vi "test_Packet_SimplePipelineResult.vi"(8 "error in (no error)":errorcluster) -> (0 "error out":errorcluster, 3 "Test Passed":bool)   [LabVIEW 2020]
uses:
  PhotonVisionLib/PhotonVisionLib.lvlib
  <vilib>/Rock Robotics/WPI/ThirdParty/JAS_Junk/TrajLib/Trajectory_Library.lvlib
  PhotonVisionLib/TypeDef/TargetCornerType.ctl
  <vilib>/Rock Robotics/WPI/ThirdParty/JAS_Junk/TrajLib/TypeDef/TRANSLATION2D.ctl
  <vilib>/Rock Robotics/WPI/ThirdParty/JAS_Junk/TrajLib/TypeDef/ROTATION2D.ctl
  <vilib>/Rock Robotics/WPI/ThirdParty/JAS_Junk/TrajLib/TypeDef/TRANSFORM2D.ctl
  PhotonVisionLib/TypeDef/PhotonTrackedTargetType.ctl
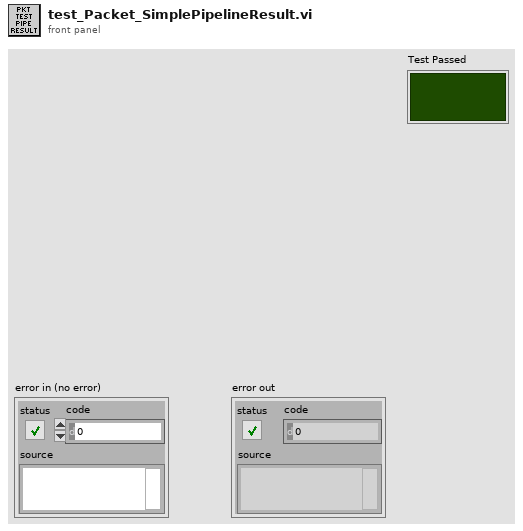
[diagram p1: front panel]
types:
  T1 = typedef "PhotonVisionLib.lvlib/PhotonTrackedTargetType.ctl" = cluster{"Yaw":dbl, "Pitch":dbl, "Area":dbl, "Skew":dbl, "TargetCorners":T2[], "CameraToTarget":T3, "FiducialId":i32}
  T2 = typedef "PhotonVisionLib.lvlib/TargetCornerType.ctl" = cluster{"X":dbl, "Y":dbl}
  T3 = typedef "Trajectory_Library.lvlib/TRANSFORM2D.ctl" = cluster{"TRANSLATION":T4, "ROTATION":T5, "xF":bool}
  T4 = typedef "Trajectory_Library.lvlib/TRANSLATION2D.ctl" = cluster{"X":dbl, "Y":dbl}
  T5 = typedef "Trajectory_Library.lvlib/ROTATION2D.ctl" = cluster{"VALUE":dbl, "COS":dbl, "SIN":dbl}
  T6 = typedef "PhotonVisionLib.lvlib/PhotonPipelineResultType.ctl" = cluster{"TargetCount":i32, "Latency_MilliSec":dbl, "Targets":T1[]}
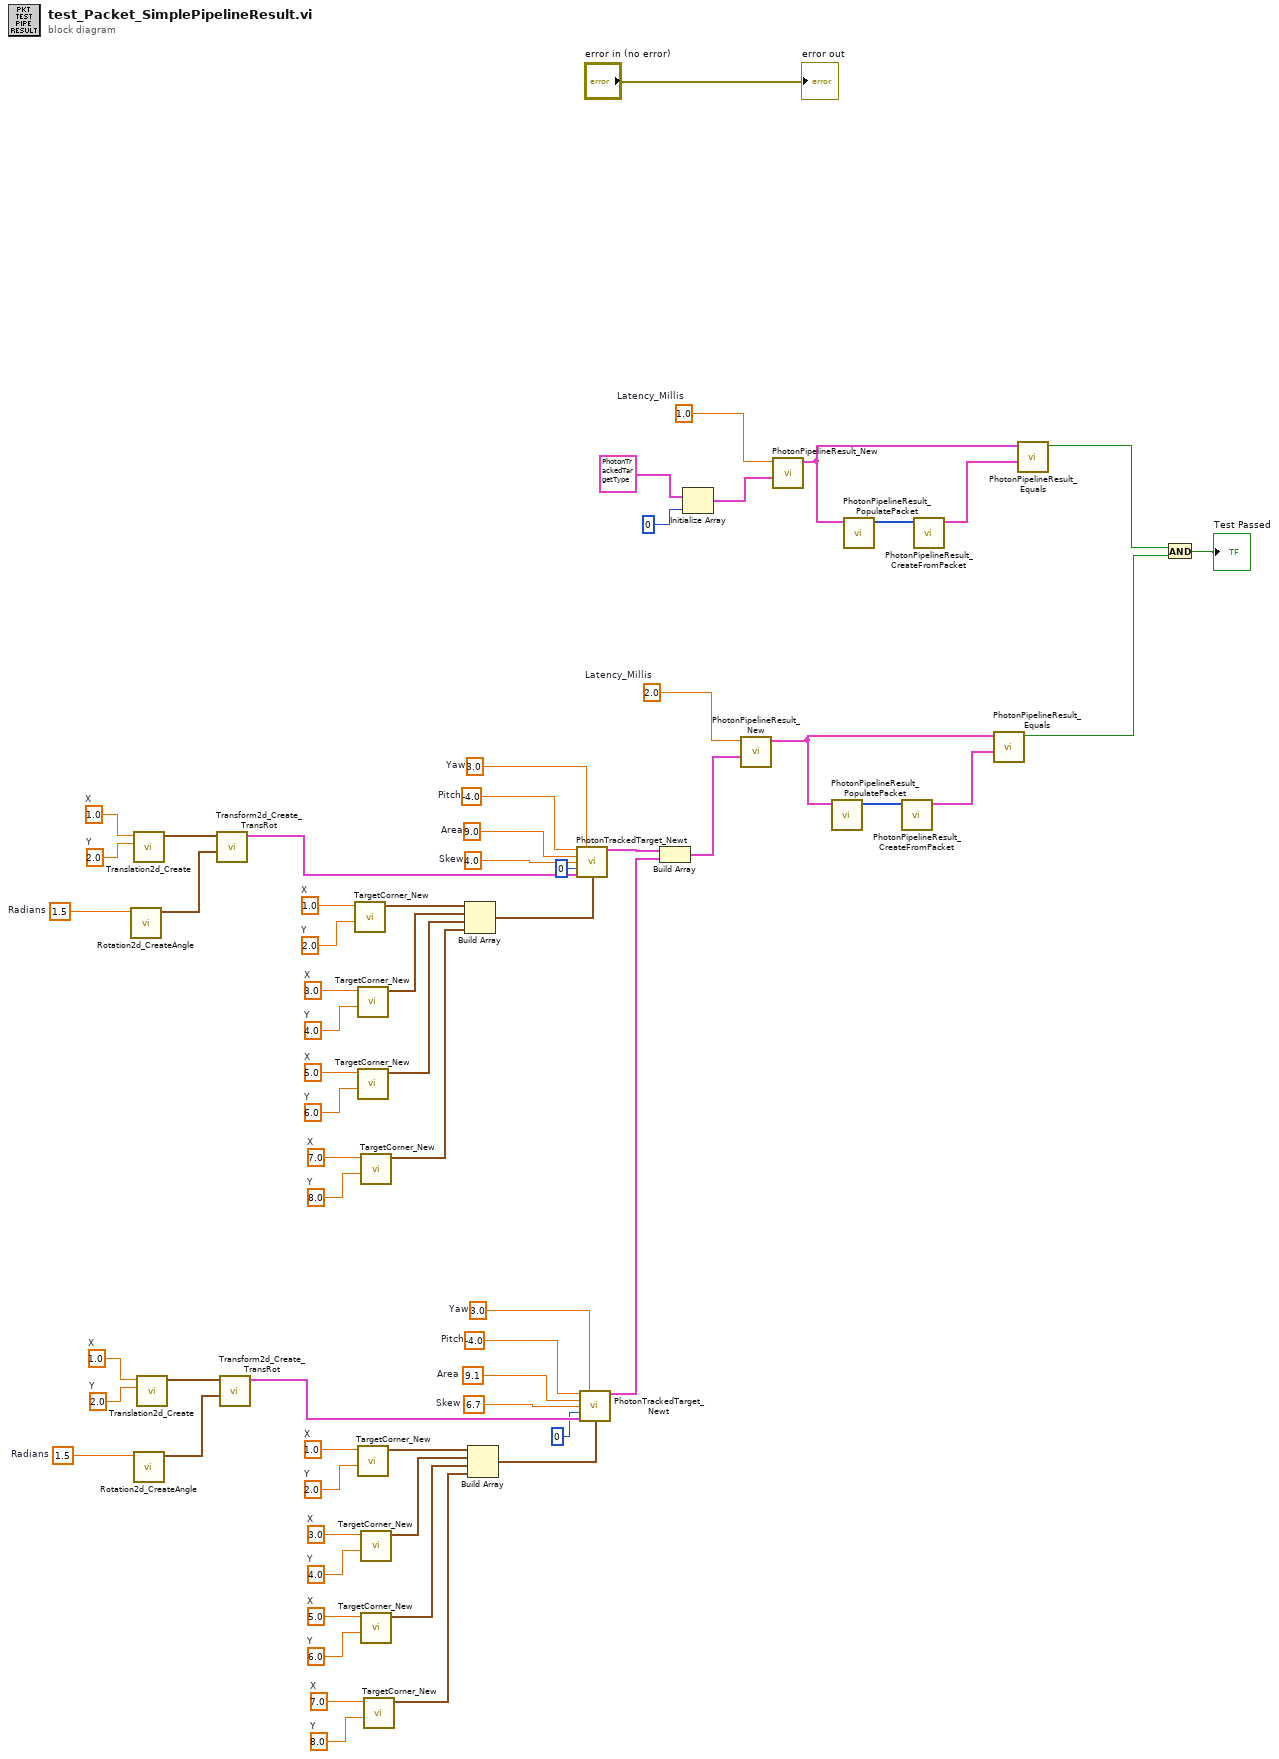
[diagram p0: block diagram]
diagram:
  w14 = 1.0  # Latency_Millis
  w16 = 2.0  # Latency_Millis
  w21 = 1.0  # X
  w22 = 2.0  # Y
  w24 = 1.5  # Radians
  w26 = -4.0  # Pitch
  w27 = 9.1  # Area
  w28 = 6.7  # Skew
  w29 = 3.0  # Yaw
  w35 = 7.0  # X
  w36 = 8.0  # Y
  w37 = 5.0  # X
  w38 = 6.0  # Y
  w39 = 3.0  # X
  w40 = 4.0  # Y
  w41 = 1.0  # X
  w42 = 2.0  # Y
  w44 = 1.0  # X
  w45 = 2.0  # Y
  w47 = 1.5  # Radians
  w49 = -4.0  # Pitch
  w50 = 9.0  # Area
  w51 = 4.0  # Skew
  w52 = 3.0  # Yaw
  w58 = 7.0  # X
  w59 = 8.0  # Y
  w60 = 5.0  # X
  w61 = 6.0  # Y
  w62 = 3.0  # X
  w63 = 4.0  # Y
  w64 = 1.0  # X
  w65 = 2.0  # Y
  n1 = call <vilib>:"Rotation2d_CreateAngle.vi"("Angle"=w47) -> ("ROTATION"=w46:T5)  [unwired: 10 in]
  n2 = call <vilib>:"Translation2d_Create.vi"("Y"=w45, "X"=w44) -> ("TRANSLATION"=w48:T4)  [unwired: 9 in]
  n3 = call <vilib>:"Rotation2d_CreateAngle.vi"("Angle"=w24) -> ("ROTATION"=w23:T5)  [unwired: 10 in]
  n4 = call <vilib>:"Translation2d_Create.vi"("Y"=w22, "X"=w21) -> ("TRANSLATION"=w25:T4)  [unwired: 9 in]
  n5 = call <vilib>:"Transform2d_Create_TransRot.vi"("ROTATION"=w46, "TRANSLATION"=w48) -> ("TRANSFORM"=w43:T3)  [unwired: 9 in]
  n6 = call <vilib>:"Transform2d_Create_TransRot.vi"("ROTATION"=w23, "TRANSLATION"=w25) -> ("TRANSFORM"=w20:T3)  [unwired: 9 in]
  n7 = call "TargetCorner_New.vi"("Y"=w65, "X"=w64) -> ("TargetCorner"=w57:T2)  [unwired: 9 in]
  n8 = call "TargetCorner_New.vi"("Y"=w63, "X"=w62) -> ("TargetCorner"=w55:T2)  [unwired: 9 in]
  n9 = call "TargetCorner_New.vi"("Y"=w61, "X"=w60) -> ("TargetCorner"=w54:T2)  [unwired: 9 in]
  n10 = call "TargetCorner_New.vi"("Y"=w42, "X"=w41) -> ("TargetCorner"=w34:T2)  [unwired: 9 in]
  n11 = call "TargetCorner_New.vi"("Y"=w59, "X"=w58) -> ("TargetCorner"=w53:T2)  [unwired: 9 in]
  n12 = call "TargetCorner_New.vi"("Y"=w40, "X"=w39) -> ("TargetCorner"=w32:T2)  [unwired: 9 in]
  n13 = call "TargetCorner_New.vi"("Y"=w38, "X"=w37) -> ("TargetCorner"=w31:T2)  [unwired: 9 in]
  n14 = call "TargetCorner_New.vi"("Y"=w36, "X"=w35) -> ("TargetCorner"=w30:T2)  [unwired: 9 in]
  n15 = Build Array(w57, w55, w54, w53) -> (w56:T2[])
  n16 = Build Array(w34, w32, w31, w30) -> (w33:T2[])
  n17 = call "PhotonTrackedTarget_Newt.vi"("Pitch"=w49, "Yaw"=w52, "Area"=w50, "Skew"=w51, "FiducalId"=0, "CameraToTarget"=w43, "TargetCorners"=w56) -> ("TrackedTarget"=w19:T1)  [unwired: 8 in]
  n18 = call "PhotonTrackedTarget_Newt.vi"("Pitch"=w26, "Yaw"=w29, "Area"=w27, "Skew"=w28, "FiducalId"=0, "CameraToTarget"=w20, "TargetCorners"=w33) -> ("TrackedTarget"=w18:T1)  [unwired: 8 in]
  n19 = Build Array(w19, w18) -> (w17:T1[])
  n20 = Initialize Array(T1 {"Yaw"=0.0, "Pitch"=0.0, "Area"=0.0, "Skew"=0.0, "TargetCorners"=[], "CameraToTarget"={"TRANSLATION"={"X"=0.0, "Y"=0.0}, "ROTATION"={"VALUE"=0.0, "COS"=1.0, "SIN"=0.0}, "xF"=FALSE}, "FiducialId"=0} ("PhotonTrackedTarget"), 0 ("dimension size")) -> (w11:T1[])
  n21 = call "PhotonPipelineResult_New.vi"("TrackedTargets"=w17, "Latency_Millis"=w16) -> ("PhotonPipelineResult"=w7:T6)  [unwired: 9 in]
  n22 = call "PhotonPipelineResult_New.vi"("TrackedTargets"=w11, "Latency_Millis"=w14) -> ("PhotonPipelineResult"=w9:T6)  [unwired: 9 in]
  n23 = call "PhotonPipelineResult_PopulatePacket.vi"("PhotonPipelineResult"=w7) -> ("Packet_RawData"=w15:u8[])  [unwired: 10 in]
  n24 = call "PhotonPipelineResult_PopulatePacket.vi"("PhotonPipelineResult"=w9) -> ("Packet_RawData"=w10:u8[])  [unwired: 10 in]
  n25 = call "PhotonPipelineResult_CreateFromPacket.vi"("RawData"=w15) -> ("PhotonPipelineResult"=w6:T6)  [unwired: 10 in]
  n26 = call "PhotonPipelineResult_CreateFromPacket.vi"("RawData"=w10) -> ("PhotonPipelineResult"=w8:T6)  [unwired: 10 in]
  n27 = call "PhotonPipelineResult_Equals.vi"("Other PhotonPipelineResult"=w6, "PhotonPipelineResult"=w7) -> ("Equal"=w3:bool)  [unwired: 9 in]
  n28 = call "PhotonPipelineResult_Equals.vi"("Other PhotonPipelineResult"=w8, "PhotonPipelineResult"=w9) -> ("Equal"=w4:bool)  [unwired: 9 in]
  n29 = And(x=w4, y=w3) -> (x .and. y?=→"Test Passed":bool)
  "error out" <- "error in (no error)"
